vi "open.vi"() -> (2 "w":i32, 3 "SystemIdVarPtr":refnum<k24>, 4 "ContextAppVarPtr":refnum<k24>, 6 "h":i32, 8 "DisplayIdVarPtr":refnum<k24>, 10 "DigitizerIdVarPtr":refnum<k24>, 13 "Mbuf":refnum<k24>, 14 "new reference":refnum<k24>, 15 "error out":errorcluster)   [LabVIEW 2019]
uses:
  C:/Users/huang/Desktop/MIL LITE 10/64/Matrox Imaging/MIL/MIL.NET/Matrox.MatroxImagingLibrary.v3.5.dll
  64/Matrox Imaging/MIL/MIL.NET/Matrox.MatroxImagingLibrary.v3.5.dll
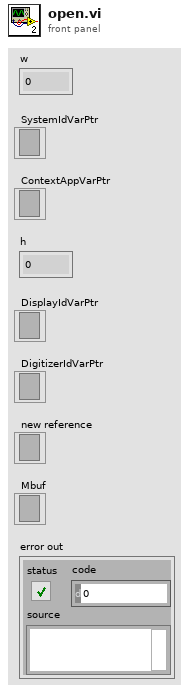
[diagram p1: front panel]
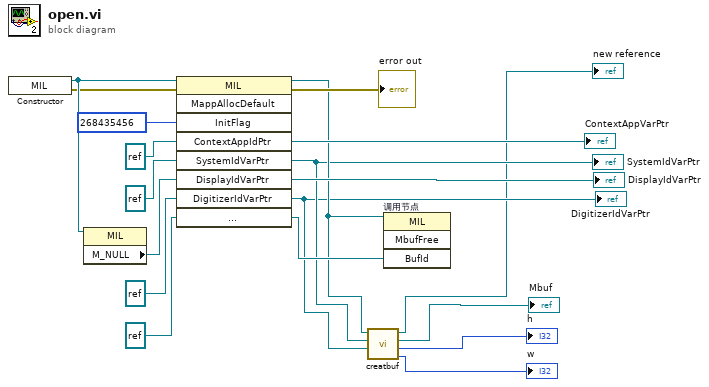
[diagram p0: block diagram]
diagram:
  n1 = constructor class="MIL"() -> (reference out=w16:refnum<k24>, error out=w15:errorcluster)  [unwired: 3 in, 1 out]
  n2 = property class="MIL"(reference=w16) -> ("M_NULL"=w17:refnum<k24>)  [unwired: 1 in, 2 out]
  n3 = invoke on="调用节点" class="MIL" method="MappAllocDefault"(reference=w16, error in=w15, "InitFlag"=i64 268435456, "ContextAppIdPtr"=refnum<k24> refnum, "SystemIdVarPtr"=refnum<k24> refnum, "DisplayIdVarPtr"=w17, "DigitizerIdVarPtr"=refnum<k24> refnum, "ImageIdVarPtr"=refnum<k24> refnum) -> (reference out=w7:refnum<k24>, error out=→"error out":errorcluster, "ContextAppIdPtr"=→"ContextAppVarPtr":refnum<k24>, "SystemIdVarPtr"=w6:refnum<k24>, "DisplayIdVarPtr"=→"DisplayIdVarPtr":refnum<k24>, "DigitizerIdVarPtr"=w5:refnum<k24>, "ImageIdVarPtr"=w18:refnum<k24>)  [unwired: 1 in, 2 out]
  "DigitizerIdVarPtr" <- w5
  "SystemIdVarPtr" <- w6
  n4 = call "creatbuf.vi"("DigitizerIdVarPtr"=w5, "SystemIdVarPtr"=w6, ".NET  in"=w7) -> ("w"=→"w":i32, "h"=→"h":i32, "MbufAlloc2d"=→"Mbuf":refnum<k24>, ".NET  out"=→"new reference":refnum<k24>)  [unwired: 3 in]
  n5 = invoke on="调用节点" class="MIL" method="MbufFree"(reference=w7, "BufId"=w18) -> ()  [unwired: 2 in, 4 out]
